vi "test Get Bitrate Info.vi"(11 "Test Case In":refnum<class "Test PCANBasic.lvclass">) -> (0 "error out":errorcluster, 3 "Test Case Out":refnum<class "Test PCANBasic.lvclass">)   [LabVIEW 2020, in "Test PCANBasic.lvclass"]
uses:
  Test PCANBasic.lvclass
  Test PCANBasic.lvclass/Test PCANBasic.ctl
  source/PCANBasic.lvlib
  source/PCAN Baud.ctl
  <vilib>/Astemes/LUnit/Test Case.lvclass
  Global PCAN Channel.vi
  source/Get Bitrate Info.vi
  Global PCAN Baudrate.vi
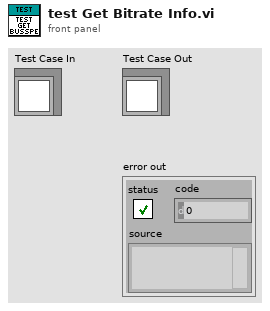
[diagram p1: front panel]
types:
  T1 = typedef "PCANBasic.lvlib/PCAN Baud.ctl" = u16
  T2 = typedef "PCANBasic.lvlib/TPCANHandle.ctl" = u16
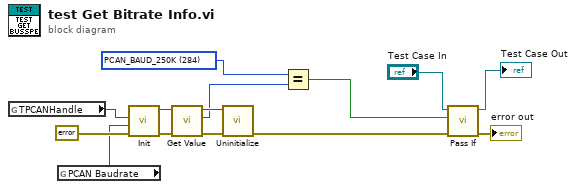
[diagram p0: block diagram]
diagram:
  w2 = T1 284 items=["PCAN_BAUD_1M"=20, "PCAN_BAUD_800K"=22, "PCAN_BAUD_500K"=28, "PCAN_BAUD_250K"=284, "PCAN_BAUD_125K"=796, "PCAN_BAUD_100K"=17199, "PCAN_BAUD_95K"=49998, "PCAN_BAUD_83K"=34091, "PCAN_BAUD_50K"=18223, "PCAN_BAUD_47K"=5140, "PCAN_BAUD_33K"=35631, "PCAN_BAUD_20K"=21295, "PCAN_BAUD_10K"=26415, "PCAN_BAUD_5K"=32639] ("Baudrate")
  n1 = global read "Global PCAN Channel.vi" "TPCANHandle"() -> (w8:T2)
  n2 = global read "Global PCAN Baudrate.vi" "PCAN Baudrate"() -> (w6:T1)
  n3 = call "Init.vi"("error in"=errorcluster {"status"=FALSE, "code"=0, "source"=""}, "Baudrate"=w6, "Channel"=w8) -> ("error out"=w9:errorcluster, "TPCANHandle out"=w7:T2)  [unwired: 6 in, 1 out]
  n4 = call-poly "Get Value.vi"("error in"=w9, "TPCANHandle in"=w7) -> ("error out"=w11:errorcluster, "Baudrate"=w1:T1, "TPCANHandle out"=w4:T2)  [unwired: 6 in, 1 out]
  n5 = call "Uninitialize.vi"("error in"=w11, "TPCANHandle in"=w4) -> ("error out"=w5:errorcluster)  [unwired: 8 in, 1 out]
  n6 = Equal?(x=w2, y=w1) -> (x = y?=w3:bool)
  n7 = call <vilib>:"Pass If.vi"("error in (no error)"=w5, "Pass?"=w3, "LUnit Test Case In"="Test Case In") -> ("error out"=→"error out":errorcluster, "LUnit Test Case Out"=→"Test Case Out":refnum<class "Test PCANBasic.lvclass">)  [unwired: 7 in]
